vi "RTI Connext DDS Secure Shapes Writer.vi"() -> ()   [LabVIEW 2012]
doc: "Shows how to publish to an existing DDS application, RTI Shapes Demo. It was created using the Tutorial of the Getting Started Guide (<LabVIEW folder>/help/RTI DDS Toolkit for LabVIEW/RTI_DDS_Toolkit_for_LabVIEW_GettingStarted.pdf)."
uses:
  RTI/GIT_HEAD/connextdds/lvdds.1.0/srcLV/lvdds.1.0_package/Types/RTI DDS Advanced Writer Configuration.ctl
  RTI/GIT_HEAD/connextdds/lvdds.1.0/srcLV/lvdds.1.0_package/Types/RTI DDS Security Settings.ctl
  RTI/GIT_HEAD/connextdds/lvdds.1.0/srcLV/lvdds.1.0_package/Types/RTI DDS Basic Security Settings.ctl
  RTI/GIT_HEAD/connextdds/lvdds.1.0/srcLV/lvdds.1.0_package/Types/RTI DDS Advanced Security Settings.ctl
  RTI/GIT_HEAD/connextdds/lvdds.1.0/srcLV/lvdds.1.0_package/Examples/ShapesDemo/RTI Connext DDS Shape Type.ctl
  RTI/GIT_HEAD/connextdds/lvdds.1.0/srcLV/lvdds.1.0_package/Library/LVDDS_library.lvlib
  RTI/GIT_HEAD/connextdds/lvdds.1.0/lib/rtilvdds.dll
panel:
  in  "Topic Name":string(combo)="Square"
  in  "Domain Id":u32
  in  "Advanced Writer Configuration":T1
  in  "error in (no error)":errorcluster
  in  "Offset y":dbl=125.0 min=0.0 max=250.0 step=2.0
  in  "Offset x":dbl=110.0 min=0.0 max=220.0 step=2.0
  in  "Frequency":dbl(knob)=0.6461186004004856 min=0.0 max=1.0 step=0.05 scale=0.0..1.0
  in  "Amplitude y":dbl(slide)=44.89795918367347 min=0.0 max=100.0 step=5.0 scale=0.0..100.0
  in  "Amplitude x":dbl(slide)=38.14432989690721 min=0.0 max=100.0 step=5.0 scale=0.0..100.0
  in  "color":string="BLUE"
  in  "shapesize":i32=25
  out "y":i32
  out "x":i32
  in  "Stop":bool
  # "This Example will show Security capabilities using RTI Shapes Demo example. \n\nRTI Shapes Demo is a sample application that demonstrates DDS concepts. It publishes and subscribes to data of type “ShapeType”, which consists of color, x and y coordinates, and a shape size. You can use this example VI to publish ShapeType data using RTI Connext DDS. You can display the data by running RTI Shapes Demo and subscribing to the corresponding topic or using Secure Shapes Reader.vi."
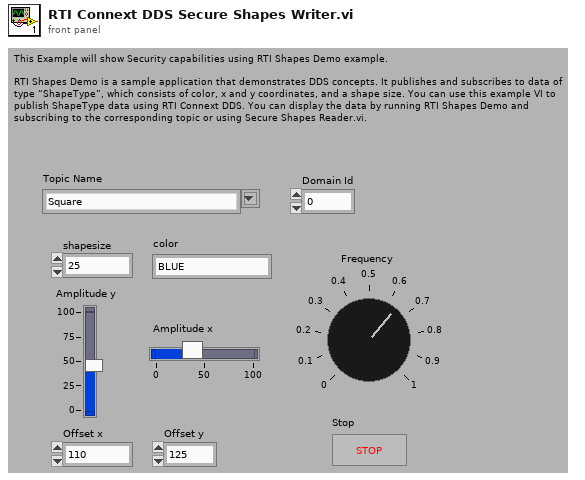
[diagram p1: front panel]
types:
  T1 = typedef "LVDDS_library.lvlib/RTI DDS Advanced Writer Configuration.ctl" = cluster{"typeName":string, "keyName":string, "domainParticipantQoSProfile":string, "dataWriterQoSProfile":string, "forceNewDomainParticipant?":bool, "forceArrayMapping?":bool, "forceUnboundedString?":bool}
  T2 = typedef "LVDDS_library.lvlib/RTI DDS Security Settings.ctl" = cluster{"Basic Security Settings":T3, "Advanced Security Settings":T4}
  T3 = typedef "LVDDS_library.lvlib/RTI DDS Basic Security Settings.ctl" = cluster{"Identity Certificate Authority (CA)":path, "Identity Certificate (Signed by Identity CA)":path, "Private Key":path, "Permissions Certificate Authority (CA)":path, "Governance Document (Signed by Permissions CA)":path, "Permissions Document (Signed by Permissions CA)":path}
  T4 = typedef "LVDDS_library.lvlib/RTI DDS Advanced Security Settings.ctl" = cluster{"Shared Secret Algorithm":string, "Encryption Algorithm":string, "Certificate Revocation List":path}
  T5 = typedef "RTI Connext DDS Shape Type.ctl" = cluster{"color":string, "x":i32, "y":i32, "shapesize":i32}
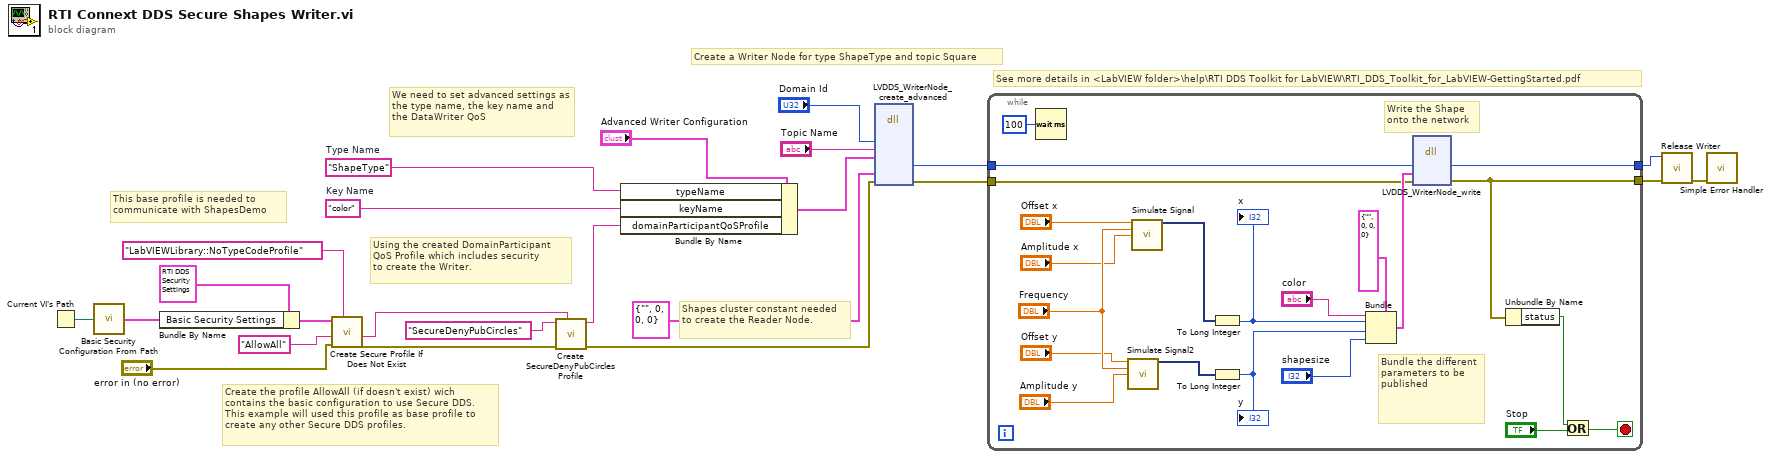
[diagram p0: block diagram]
diagram:
  w17 = "color"  # Key Name
  w16 = "ShapeType"  # Type Name
  # "Create the profile AllowAll (if doesn't exist) wich \ncontains the basic configuration to use Secure DDS.\nThis example will used this profile as base profile to \ncreate any other Secure DDS profiles."
  # "This base profile is needed to \ncommunicate with ShapesDemo"
  # "Using the created DomainParticipant \nQoS Profile which includes security \nto create the Writer."
  # "We need to set advanced settings as the type name, the key name and the DataWriter QoS"
  # "See more details in <LabVIEW folder>\\help\\RTI DDS Toolkit for LabVIEW\\RTI_DDS_Toolkit_for_LabVIEW-GettingStarted.pdf"
  # "Shapes cluster constant needed to create the Reader Node."
  # "Create a Writer Node for type ShapeType and topic Square"
  n1 = Current VI's Path() -> (path=w6:path)
  n2 = call "Basic Security Configuration From Path.vi"("Current Path"=w6) -> ("Basic Security Settings"=w9:T3)
  n3 = Bundle By Name(cluster=T2 {"Basic Security Settings"={"Identity Certificate Authority (CA)"=path "", "Identity Certificate (Signed by Identity CA)"=path "", "Private Key"=path "", "Permissions Certificate Authority (CA)"=path "", "Governance Document (Signed by Permissions CA)"=path "", "Permissions Document (Signed by Permissions CA)"=path ""}, "Advanced Security Settings"={"Shared Secret Algorithm"="ecdsa-ecdh", "Encryption Algorithm"="aes-128-gcm", "Certificate Revocation List"=path ""}} ("Security Settings"), "Basic Security Settings"=w9) -> (w8:T2)
  n4 = call "Create Secure Profile If Does Not Exist.vi"("Base Profile"="LabVIEWLibrary::NoTypeCodeProfile", "error in (no error)"="error in (no error)", "New Profile Name"="AllowAll", "Security Settings"=w8) -> ("error out"=w4:errorcluster, "New Profile Name Output"=w2:string)  [unwired: 6 in]
  n5 = call "Create SecureDenyPubCircles Profile.vi"("DomainParticipant Base Profile Name"=w2, "error in (no error)"=w4, "New Custom Secure Profile Name"="SecureDenyPubCircles") -> ("error out"=w3:errorcluster, "Custom Secure Profile Name Output"=w1:string)  [unwired: 7 in]
  n6 = Bundle By Name(cluster="Advanced Writer Configuration", "typeName"=w16, "keyName"=w17, "domainParticipantQoSProfile"=w1) -> (w15:T1)
  n7 = dll-call lib="D:/RTI/GIT_HEAD/connextdds/lvdds.1.0/lib/rtilvdds.*" fn="LVDDS_WriterNode_create_advanced"("domain id"="Domain Id", "topic name"="Topic Name", "advanced writer configuration"=w15, "data type"=T5 {"color"="", "x"=0, "y"=0, "shapesize"=0} ("Shape"), w3) -> ("ref num"=w21:u64, w20:errorcluster)  [unwired: 11 in, 2 out]
  n8 = while {
    tunnel: w21 -> [w45]
    tunnel: [w44] -> w24
    tunnel: w20 -> [w30]
    tunnel: [w26] -> w23
    stop <- w25 stop-if-true
    # "Bundle the different parameters to be published"
    # "Write the Shape \nonto the network"
    n9 = Wait (ms)(milliseconds to wait=u32 100) -> ()  [unwired: 1 out]
    n10 = call "Simulate Signal2"("Offset"="Offset y", "Frequency"="Frequency", "Amplitude"="Amplitude y") -> ("Sine"=w35:dynamicdata)  [unwired: 11 in, 1 out]
    n11 = call "Simulate Signal"("Offset"="Offset x", "Frequency"="Frequency", "Amplitude"="Amplitude x") -> ("Sine"=w34:dynamicdata)  [unwired: 11 in, 1 out]
    n12 = To Long Integer(number=w34) -> (32bit integer=w36:i32)
    "x" <- w36
    n13 = To Long Integer(number=w35) -> (32bit integer=w38:i32)
    "y" <- w38
    n14 = Bundle(cluster=T5 {"color"="", "x"=0, "y"=0, "shapesize"=0} ("Shape"), "color"="color", "x"=w36, "y"=w38, "shapesize"="shapesize") -> (w31:T5)
    n15 = dll-call lib="D:/RTI/GIT_HEAD/connextdds/lvdds.1.0/lib/rtilvdds.dll" fn="LVDDS_WriterNode_write"("Ref Num"=w45, "Shape"=w31, "Error"=w30) -> ("Ref Num"=w44:u64, "Error"=w26:errorcluster)  [unwired: 5 in, 2 out]
    n16 = Unbundle By Name(w26) -> ("status"=w28:bool)
    n17 = Or(x=w28, y="Stop") -> (x .or. y?=w25:bool)
  }
  n18 = call "Release Writer.vi"("error in"=w23, "ref num"=w24) -> ("error out"=w22:errorcluster)  [unwired: 9 in]
  n19 = call <vilib>:"Simple Error Handler.vi"("error in (no error)"=w22) -> ()  [unwired: 4 in, 5 out]
